vi "Create mailboxes.vi"(4 "error in (no error)":errorcluster, 5 "max queue size (-1, unlimited)":i32, 7 "List of names (empty)":string[](array[string])) -> (0 "error out":errorcluster, 1 "created new?":bool[](array[boolean]), 3 "Mailboxes":T1)   [LabVIEW 2021, in "MatS Libs.lvlib"]
doc: "Creates mailboxes for given list (array) of names, and outputs them as a collection (map/dictionary). \nIf mailbox with given name already exist it is not created, but its reference is also obtained and add to collection (see \"created new?\" array)."
uses:
  <userlib>/MatS Libs/MatS Mailman/TypeDefs/Mailboxes.ctl
  <userlib>/MatS Libs/MatS Mailman/TypeDefs/Mailbox ref.ctl
  <userlib>/MatS Libs/MatS Libs.lvlib
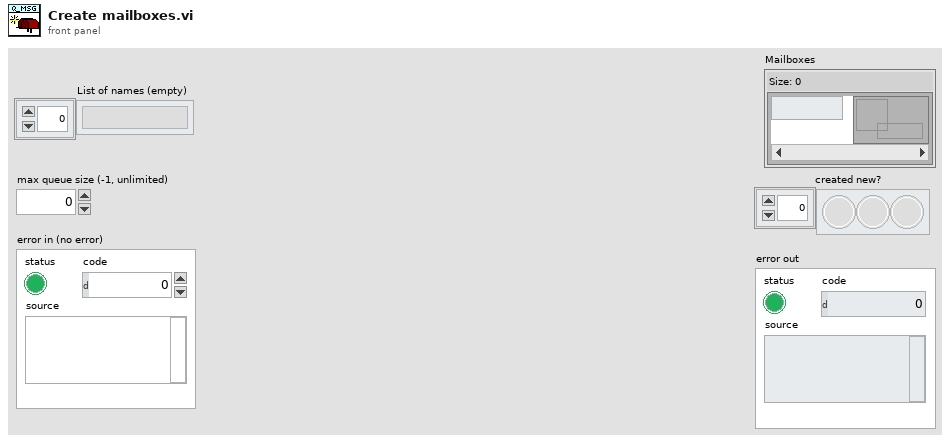
[diagram p1: front panel]
types:
  T1 = typedef "MatS Libs.lvlib/Mailboxes.ctl" = map{string, T2}
  T2 = typedef "MatS Libs.lvlib/Mailbox ref.ctl" = refnum<queue>
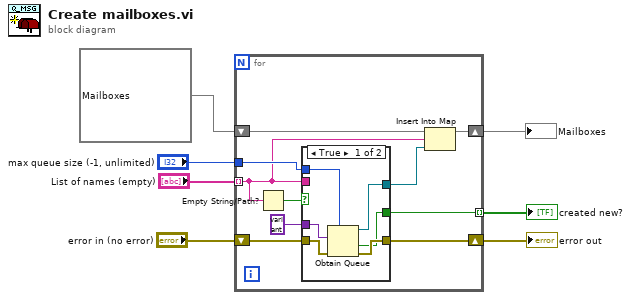
[diagram p0: block diagram]
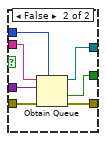
[diagram p2: hidden frame]
diagram:
  n1 = for {
    tunnel: "max queue size (-1, unlimited)" -> [w17]
    tunnel: [w14] -> w4 mode=indexing
    tunnel: "List of names (empty)" -> [w11] mode=indexing
    shift-right: [w15] -> w5
    shift-left: "error in (no error)" -> [w16]
    shift-right: [w10] -> w1
    shift-left: T1 {} -> [w8]
    n2 = Empty String/Path?(string/path=w11) -> (empty?=w13:bool)
    n3 = case shown="True" w13 {
      tunnel: variant -> [w18 w30]
      tunnel: w17 -> [w23 w29]
      tunnel: w11 -> [_ w28]
      tunnel: w16 -> [w22 w27]
      tunnel: [w21 w26] -> w15
      tunnel: [w20 w25] -> w14
      tunnel: [w19 w24] -> w9
      frame True {
        n4 = Obtain Queue(max queue size (-1, unlimited)=w23, element data type=w18, error in (no error)=w22) -> (queue out=w19:refnum<queue>, created new?=w20:bool, error out=w21:errorcluster)  [unwired: 2 in]
      }
      frame False {
        n5 = Obtain Queue(max queue size (-1, unlimited)=w29, name (unnamed)=w28, element data type=w30, error in (no error)=w27) -> (queue out=w24:refnum<queue>, created new?=w25:bool, error out=w26:errorcluster)  [unwired: 1 in]
      }
    }
    n6 = Insert Into Map(map in=w8, key=w11, value=w9) -> (map out=w10:T1)  [unwired: 2 out]
  }
  "error out" <- w5
  "created new?" <- w4
  "Mailboxes" <- w1
